vi "Tree Empty.vi"(0 "Tree Reference In":refnum<vi>, 5 "error in (no error)":errorcluster, 8 "Return Elements (f)":bool) -> (14 "Tree Reference Out":refnum<vi>, 16 "Deleted Tree Items":string[](array[string]), 19 "error out":errorcluster)   [LabVIEW 2015, in "QuickVIew.lvlib"]
doc: "Deletes all elements from<B>Tree Reference In</B>. Passes deleted elements from the tree out in a 1-D array. The array is ordered top to bottom item as they were in the tree.TLB Prime - Application Template 1.3.0.24\nNorm Kirchner, NI Systems Engineering - NI\nCopyright (c) 2014, NI"
uses:
  QuickVIew.lvlib
  Typedef/TYPEDEF - DataStore Command.ctl
panel:
  # "VI INPUTS"
  # "VI OUTPUTS"
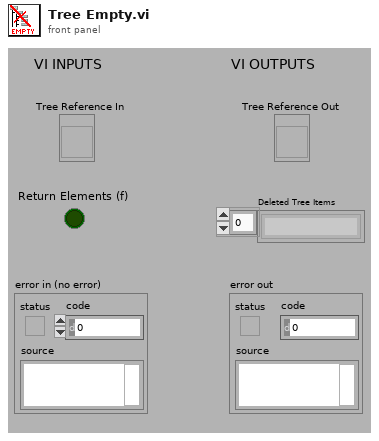
[diagram p1: front panel]
types:
  T1 = typedef "QuickVIew.lvlib/TYPEDEF - DataStore Command.ctl" = enum16{"Init", "Add", "Get", "Clear Tree", "Clear All", "Modify"}
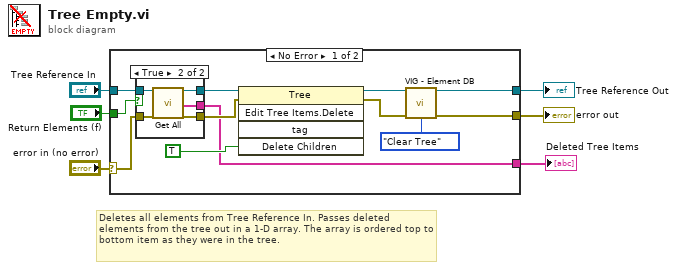
[diagram p0: block diagram]
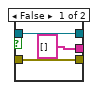
[diagram p2: hidden frame]
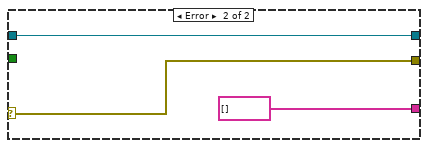
[diagram p3: hidden frame]
diagram:
  # "Deletes all elements from Tree Reference In. Passes deleted elements from the tree out in a 1-D array. The array is ordered top to bottom item as they were in the tree."
  n1 = case shown="No Error" "error in (no error)" {
    selector: "error in (no error)" -> [w17 w28]
    tunnel: "Tree Reference In" -> [w18 w29]
    tunnel: [w9 w29] -> w5
    tunnel: [w8 w28] -> w4
    tunnel: [w13 string[] []] -> w2
    tunnel: "Return Elements (f)" -> [w12 _]
    frame No Error {
      n2 = case shown="True" w12 {
        tunnel: w18 -> [w20 w26]
        tunnel: w17 -> [w21 w25]
        tunnel: [string[] [] ("Output Tree Items") w24] -> w13
        tunnel: [w20 w23] -> w16
        tunnel: [w21 w22] -> w15
        frame False {
        }
        frame True {
          n3 = call "Get All.vi"("Tree Reference In"=w26, "error in (no error)"=w25) -> ("Tree Reference Out"=w23:refnum<vi>, "Output Tree Items"=w24:string[], "error out"=w22:errorcluster)  [unwired: 15 out]
        }
      }
      n4 = invoke class="Tree" method="Edit Tree Items.Delete"(reference=w16, error in=w15, "Delete Children"=TRUE) -> (reference out=w10:refnum<vi>, error out=w11:errorcluster)  [unwired: 2 in, 3 out]
      n5 = call "VIG - Element DB.vi"("Tree Ref In"=w10, "error in (no error)"=w11, "Command"=TYPEDEF_-_DataStore_Command."Clear Tree") -> ("Tree Ref Out"=w9:refnum<vi>, "error out"=w8:errorcluster)  [unwired: 2 in, 9 out]
    }
    frame Error {
    }
  }
  "Tree Reference Out" <- w5
  "error out" <- w4
  "Deleted Tree Items" <- w2
